vi "Read Base Description.vi"(11 "Mocha in":refnum<class "Mocha.lvclass">) -> (2 "Description":string)   [LabVIEW 2013, in "Mocha.lvclass"]
uses:
  Mocha.lvclass
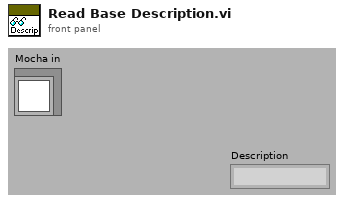
[diagram p1: front panel]
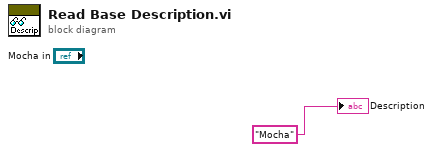
[diagram p0: block diagram]
diagram:
  "Description" <- "Mocha" ("string")
